vi "SelectRowOrCol.vi"(6 "Shift Pressed? (F)":bool, 7 "Row/Col":enum16{"row-wise", "col-wise"}(ring), 8 "error in":errorcluster, 9 "Table CtlRef":refnum<vi>, 10 "Button (1)":u16=1, 11 "CellPosition":T1) -> (0 "error out":errorcluster, 2 "Button":u16)   [LabVIEW 2013]
doc: "Select single row or column (choose functionality with row/col enum) when Shift Pressed? is false. Use Shift to make multi-row/col selection.\n\nThis VI assumes the caller has already determined the click is a row/column header (i.e. col/row in CellPosition will be <0!)"
uses:
  <vilib>/Utility/miscctls.llb/LVRowAndColumnTypeDef.ctl
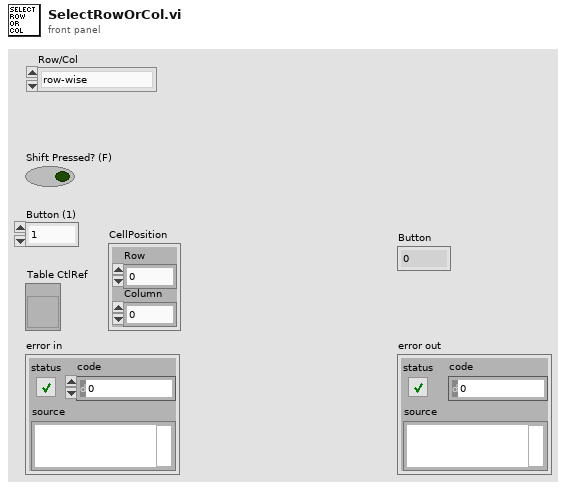
[diagram p1: front panel]
types:
  T1 = typedef "LVRowAndColumnTypeDef.ctl" = cluster{"Row":i32, "Column":i32}
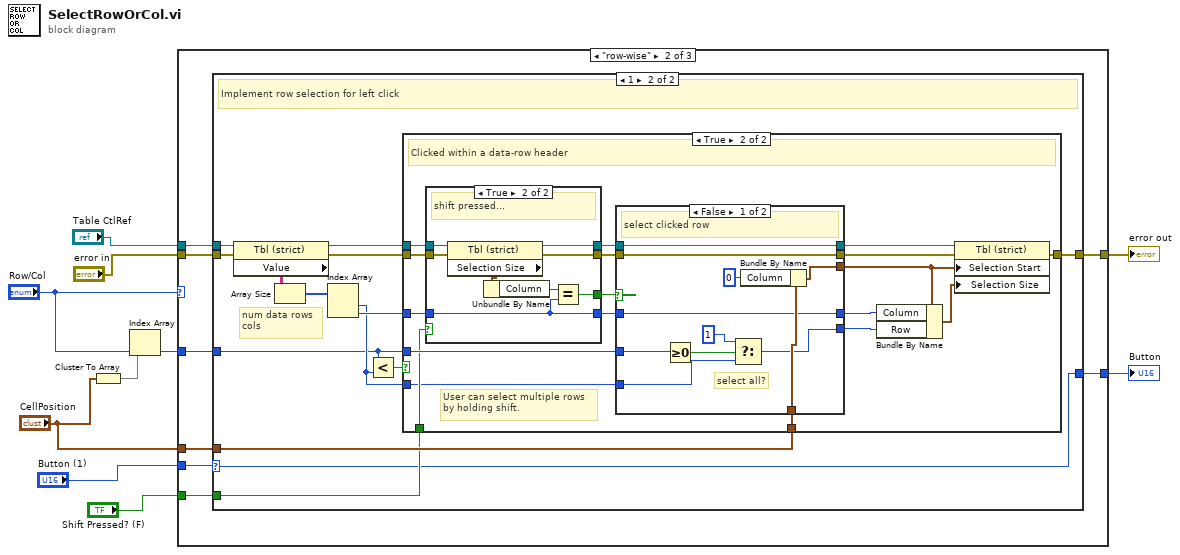
[diagram p0: block diagram]
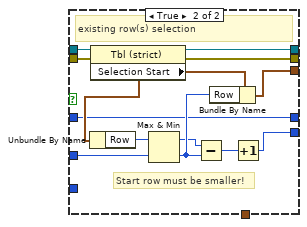
[diagram p5: hidden frame]
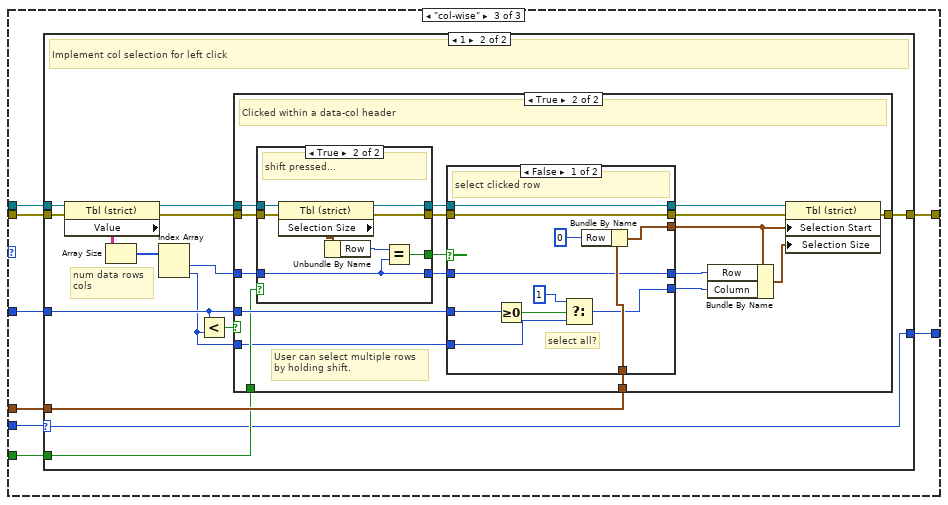
[diagram p7: hidden frame]
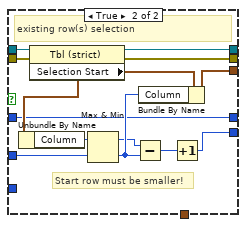
[diagram p10: hidden frame]
diagram:
  n1 = Cluster To Array(cluster="CellPosition") -> (array=w2:i32[])
  n2 = Index Array(array=w2, index="Row/Col") -> (element=w3:i32)
  n3 = case shown="\"row-wise\"" "Row/Col" {
    tunnel: "Button (1)" -> [w11 w20 w99]
    tunnel: "Shift Pressed? (F)" -> [_ w19 w98]
    tunnel: "Table CtlRef" -> [_ w18 w97]
    tunnel: "error in" -> [w12 w17 w96]
    tunnel: [w12 w16 w95] -> w6
    tunnel: [w11 w15 w94] -> w5
    tunnel: "CellPosition" -> [_ w14 w93]
    tunnel: w3 -> [_ w13 w92]
    frame Default {
    }
    frame "row-wise" {
      n4 = case shown="1" w20 {
        selector: w20 -> [w21 w27]
        tunnel: [w22 w36] -> w16
        tunnel: w17 -> [w22 w35]
        tunnel: w18 -> [_ w34]
        tunnel: w13 -> [_ w24]
        tunnel: w14 -> [_ w29]
        tunnel: w19 -> [_ w28]
        tunnel: [w21 w27] -> w15
        frame Default {
        }
        frame 1 {
          # "num data rows\ncols"
          # "Implement row selection for left click"
          n5 = property class="Tbl (strict)"(reference=w34, error in=w35) -> (reference out=w31:refnum<vi>, error out=w30:errorcluster, "Value"=w33:string[][])
          n6 = Array Size(array=w33) -> (size(s)=w32:i32[])
          n7 = Index Array(array=w32) -> (element #1=w25:i32, element #2=w26:i32)  [unwired: 2 in]
          n8 = Less?(x=w24, y=w25) -> (x < y?=w23:bool)
          n9 = case shown="True" w23 {
            tunnel: [w37 w55] -> w36
            tunnel: w31 -> [_ w54]
            tunnel: w30 -> [w37 w53]
            tunnel: w24 -> [_ w47]
            tunnel: w29 -> [_ w46]
            tunnel: w28 -> [_ w40]
            tunnel: w25 -> [_ w39]
            tunnel: w26 -> [_ w38]
            frame False {
              # "ignore row clicks below data!"
            }
            frame True {
              # "User can select multiple rows\nby holding shift."
              # "Clicked within a data-row header"
              n10 = case shown="True" w40 {
                selector: w40 -> [w83 _]
                tunnel: w54 -> [w82 w91]
                tunnel: w53 -> [w81 w90]
                tunnel: [w81 w89] -> w50
                tunnel: [w82 w88] -> w52
                tunnel: w38 -> [w80 w84]
                tunnel: [w83 w85] -> w48
                tunnel: [w80 w84] -> w45
                frame False {
                }
                frame True {
                  # "shift pressed..."
                  n11 = property class="Tbl (strict)"(reference=w91, error in=w90) -> (reference out=w88:refnum<vi>, error out=w89:errorcluster, "Selection Size"=w87:T1)
                  n12 = Unbundle By Name(w87) -> ("Column"=w86:i32)
                  n13 = Equal?(x=w86, y=w84) -> (x = y?=w85:bool)
                }
              }
              n14 = case shown="False" w48 {
                tunnel: w52 -> [w66 w79]
                tunnel: [w66 w78] -> w51
                tunnel: w50 -> [w65 w77]
                tunnel: [w65 w76] -> w49
                tunnel: w47 -> [w60 w74]
                tunnel: [w63 w73] -> w43
                tunnel: w46 -> [w64 _]
                tunnel: w45 -> [w61 w68]
                tunnel: [w61 w68] -> w44
                tunnel: [w58 w67] -> w41
                tunnel: w39 -> [w56 _]
                frame False {
                  # "select all?"
                  # "select clicked row"
                  n15 = Greater Or Equal To 0?(x=w60) -> (x >= 0?=w59:bool)
                  n16 = Select(t=1, s=w59, f=w56) -> (s? t:f=w58:i32)
                  n17 = Bundle By Name(cluster=w64, "Column"=0) -> (w63:T1)
                }
                frame True {
                  # "Start row must be smaller!"
                  # "existing row(s) selection"
                  n18 = property class="Tbl (strict)"(reference=w79, error in=w77) -> (reference out=w78:refnum<vi>, error out=w76:errorcluster, "Selection Start"=w69:T1)
                  n19 = Unbundle By Name(w69) -> ("Row"=w75:i32)
                  n20 = Max & Min(x=w75, y=w74) -> (max(x,y)=w71:i32, min(x,y)=w72:i32)
                  n21 = Subtract(x=w71, y=w72) -> (x-y=w70:i32)
                  n22 = Bundle By Name(cluster=w69, "Row"=w72) -> (w73:T1)
                  n23 = Increment(x=w70) -> (x+1=w67:i32)
                }
              }
              n24 = Bundle By Name(cluster=w43, "Column"=w44, "Row"=w41) -> (w42:T1)
              n25 = property class="Tbl (strict)"(reference=w51, error in=w49, "Selection Start"=w43, "Selection Size"=w42) -> (error out=w55:errorcluster)  [unwired: 1 out]
            }
          }
        }
      }
    }
    frame "col-wise" {
      n26 = case shown="1" w99 {
        selector: w99 -> [w100 w106]
        tunnel: [w101 w115] -> w95
        tunnel: w96 -> [w101 w114]
        tunnel: w97 -> [_ w113]
        tunnel: w92 -> [_ w105]
        tunnel: w93 -> [_ w108]
        tunnel: w98 -> [_ w107]
        tunnel: [w100 w106] -> w94
        frame Default {
        }
        frame 1 {
          # "num data rows\ncols"
          # "Implement col selection for left click"
          n27 = property class="Tbl (strict)"(reference=w113, error in=w114) -> (reference out=w110:refnum<vi>, error out=w109:errorcluster, "Value"=w112:string[][])
          n28 = Array Size(array=w112) -> (size(s)=w111:i32[])
          n29 = Index Array(array=w111) -> (element #1=w102:i32, element #2=w103:i32)  [unwired: 2 in]
          n30 = Less?(x=w105, y=w103) -> (x < y?=w104:bool)
          n31 = case shown="True" w104 {
            tunnel: [w116 w134] -> w115
            tunnel: w110 -> [_ w133]
            tunnel: w109 -> [w116 w132]
            tunnel: w105 -> [_ w126]
            tunnel: w108 -> [_ w125]
            tunnel: w107 -> [_ w119]
            tunnel: w103 -> [_ w118]
            tunnel: w102 -> [_ w117]
            frame False {
              # "ignore row clicks below data!"
            }
            frame True {
              # "User can select multiple rows\nby holding shift."
              # "Clicked within a data-col header"
              n32 = case shown="True" w119 {
                selector: w119 -> [w162 _]
                tunnel: w133 -> [w161 w170]
                tunnel: w132 -> [w160 w169]
                tunnel: [w160 w168] -> w129
                tunnel: [w161 w167] -> w131
                tunnel: w117 -> [w159 w163]
                tunnel: [w162 w164] -> w127
                tunnel: [w159 w163] -> w124
                frame False {
                }
                frame True {
                  # "shift pressed..."
                  n33 = property class="Tbl (strict)"(reference=w170, error in=w169) -> (reference out=w167:refnum<vi>, error out=w168:errorcluster, "Selection Size"=w166:T1)
                  n34 = Unbundle By Name(w166) -> ("Row"=w165:i32)
                  n35 = Equal?(x=w165, y=w163) -> (x = y?=w164:bool)
                }
              }
              n36 = case shown="False" w127 {
                tunnel: w131 -> [w145 w158]
                tunnel: [w145 w157] -> w130
                tunnel: w129 -> [w144 w156]
                tunnel: [w144 w155] -> w128
                tunnel: w126 -> [w139 w153]
                tunnel: [w142 w152] -> w122
                tunnel: w125 -> [w143 _]
                tunnel: w124 -> [w140 w147]
                tunnel: [w140 w147] -> w123
                tunnel: [w137 w146] -> w120
                tunnel: w118 -> [w135 _]
                frame False {
                  # "select all?"
                  # "select clicked row"
                  n37 = Greater Or Equal To 0?(x=w139) -> (x >= 0?=w138:bool)
                  n38 = Select(t=1, s=w138, f=w135) -> (s? t:f=w137:i32)
                  n39 = Bundle By Name(cluster=w143, "Row"=0 ("Column")) -> (w142:T1)
                }
                frame True {
                  # "Start row must be smaller!"
                  # "existing row(s) selection"
                  n40 = property class="Tbl (strict)"(reference=w158, error in=w156) -> (reference out=w157:refnum<vi>, error out=w155:errorcluster, "Selection Start"=w148:T1)
                  n41 = Unbundle By Name(w148) -> ("Column"=w154:i32)
                  n42 = Max & Min(x=w154, y=w153) -> (max(x,y)=w150:i32, min(x,y)=w151:i32)
                  n43 = Subtract(x=w150, y=w151) -> (x-y=w149:i32)
                  n44 = Bundle By Name(cluster=w148, "Column"=w151) -> (w152:T1)
                  n45 = Increment(x=w149) -> (x+1=w146:i32)
                }
              }
              n46 = Bundle By Name(cluster=w122, "Row"=w123, "Column"=w120) -> (w121:T1)
              n47 = property class="Tbl (strict)"(reference=w130, error in=w128, "Selection Start"=w122, "Selection Size"=w121) -> (error out=w134:errorcluster)  [unwired: 1 out]
            }
          }
        }
      }
    }
  }
  "error out" <- w6
  "Button" <- w5
